vi "Read Shared Variables.vi"(10 "Shared Variables To Read in":T1, 11 "Write Values in":dbl[](array[numeric])) -> (0 "error out":errorcluster, 2 "Shared Variables To Read out":T1, 3 "Write Values out":dbl[](array[numeric]))   [LabVIEW 2012, in "Shared Variable Custom Device.lvlib"]
uses:
  Shared Variable Custom Device.lvlib
  Shared Variable/Shared Variable Cluster.ctl
  Shared Variable/Shared Variable Access.ctl
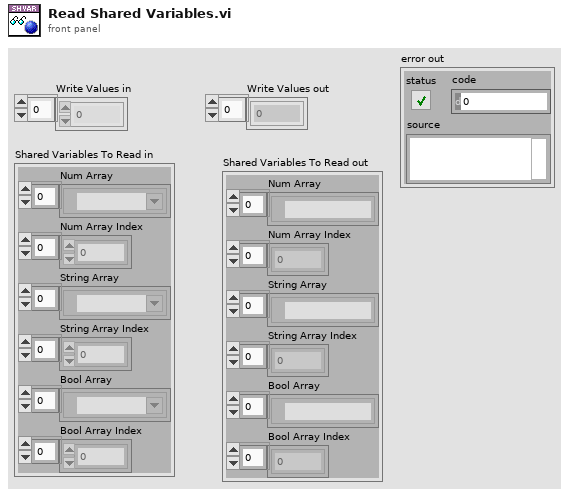
[diagram p1: front panel]
types:
  T1 = typedef "Shared Variable Custom Device.lvlib/Shared Variable Cluster.ctl" = cluster{"Num Array":refnum<k21>[], "Num Array Index":i32[], "String Array":refnum<k21>[], "String Array Index":i32[], "Bool Array":refnum<k21>[], "Bool Array Index":i32[]}
  T2 = typedef "Shared Variable Custom Device.lvlib/Shared Variable Access.ctl" = enum16{"Write", "Read"}
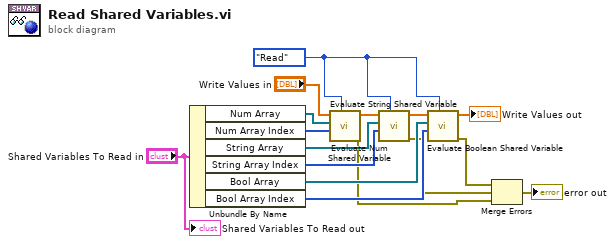
[diagram p0: block diagram]
diagram:
  w15 = Shared_Variable_Access."Read" ("Access")
  n1 = Unbundle By Name("Shared Variables To Read in") -> ("Num Array"=w6:refnum<k21>[], "Num Array Index"=w9:i32[], "String Array"=w5:refnum<k21>[], "String Array Index"=w11:i32[], "Bool Array"=w13:refnum<k21>[], "Bool Array Index"=w14:i32[])
  n2 = call "Evaluate Num Shared Variable.vi"("Access"=w15, "Num Array Index"=w9, "Num Array"=w6, "Write Values in"="Write Values in") -> ("error out"=w2:errorcluster, "Write Values out"=w10:dbl[])  [unwired: 6 in]
  n3 = call "Evaluate String Shared Variable.vi"("Access"=w15, "String Array Index"=w11, "String Array"=w5, "Write Values in"=w10) -> ("error out"=w3:errorcluster, "Write Values out"=w12:dbl[])  [unwired: 6 in]
  n4 = call "Evaluate Boolean Shared Variable.vi"("Access"=w15, "Boolean Array Index"=w14, "Boolean Array"=w13, "Write Values in"=w12) -> ("error out"=w4:errorcluster, "Write Values out"=→"Write Values out":dbl[])  [unwired: 6 in]
  n5 = Merge Errors(w4, w3, w2) -> (→"error out":errorcluster)
  "Shared Variables To Read out" <- "Shared Variables To Read in"
